vi "Read DVR.vi"(8 "error in (no error)":errorcluster, 11 "Cautious Wolf in":refnum<class "Cautious Wolf.lvclass">) -> (0 "error out":errorcluster, 2 "DVR":refnum<data-value>, 3 "Cautious Wolf out":refnum<class "Cautious Wolf.lvclass">)   [LabVIEW 2015, in "Cautious Wolf.lvclass"]
uses:
  Cautious Wolf.lvclass
  Cautious Wolf.lvclass/Cautious Wolf.ctl
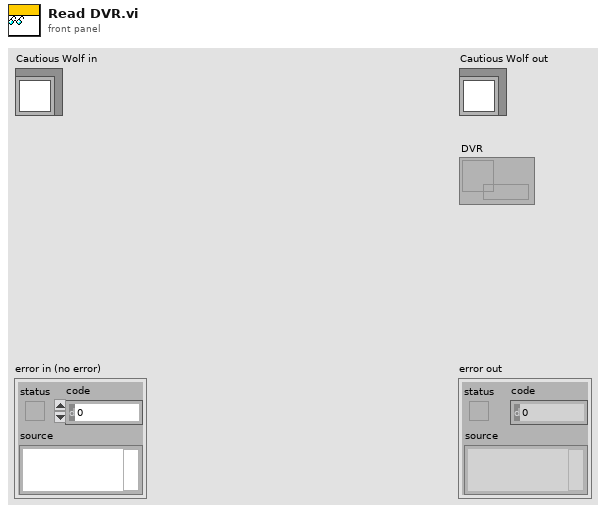
[diagram p1: front panel]
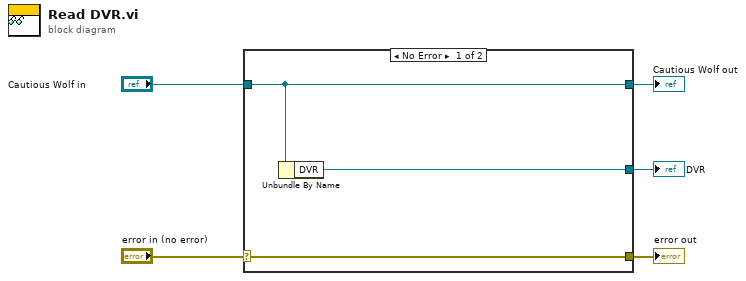
[diagram p0: block diagram]
diagram:
  n1 = case shown="No Error" "error in (no error)" {
    selector: "error in (no error)" -> [w8 w9]
    tunnel: [w8 w9] -> w4
    tunnel: [w7 w10] -> w2
    tunnel: "Cautious Wolf in" -> [w7 w10]
    tunnel: [w6 _] -> w1
    frame No Error {
      n2 = Unbundle By Name(w7) -> ("DVR"=w6:refnum<data-value>)
    }
    frame Error {
    }
  }
  "error out" <- w4
  "Cautious Wolf out" <- w2
  "DVR" <- w1
